vi "LWXPS_TZPVTExecution.vi"(0 "XPS Reference IN":refnum<k24>, 5 "TZ group name":string, 7 "Trajectory file name":string, 9 "Execution number":i32, 11 "LabVIEW error IN":errorcluster) -> (4 "XPS Reference OUT":refnum<k24>, 6 "Returned error code":i32, 8 "XPS Error String":string, 15 "LabVIEW error OUT":errorcluster)   [LabVIEW 2014]
uses:
  D:/XPSQ8_LabView_Library/Development/Source/Dll/Newport.XPS.CommandInterface.dll
  Dll/Newport.XPS.CommandInterface.dll
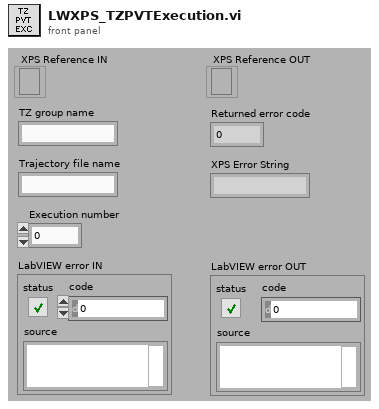
[diagram p1: front panel]
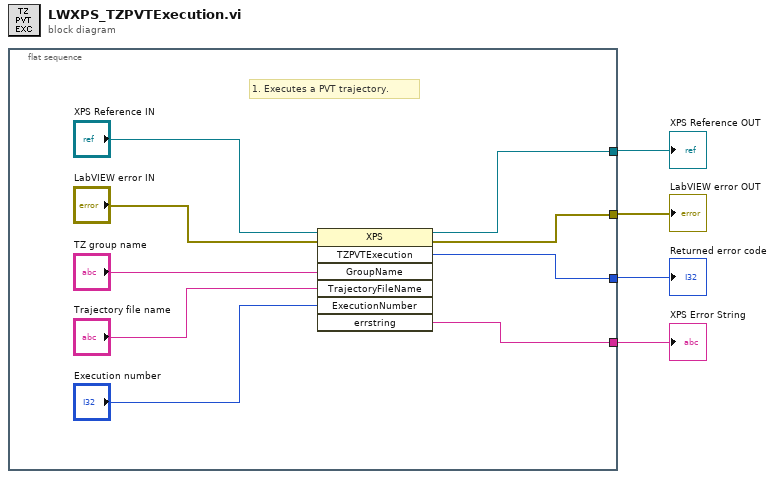
[diagram p0: block diagram]
diagram:
  n1 = flat-sequence {
    tunnel: [w9] -> w4
    tunnel: [w8] -> w3
    tunnel: [w10] -> w2
    tunnel: [w6] -> w1
    frame #0 {
      # "1. Executes a PVT trajectory."
      n2 = invoke class="XPS" method="TZPVTExecution"(reference="XPS Reference IN", error in="LabVIEW error IN", "GroupName"="TZ group name", "TrajectoryFileName"="Trajectory file name", "ExecutionNumber"="Execution number") -> (reference out=w9:refnum<k24>, error out=w8:errorcluster, "TZPVTExecution"=w10:i32, "errstring"=w6:string)  [unwired: 2 in, 3 out]
    }
  }
  "XPS Error String" <- w1
  "XPS Reference OUT" <- w4
  "LabVIEW error OUT" <- w3
  "Returned error code" <- w2
